vi "listen_can.vi"(10 "reference":refnum<vi>, 11 "队列输入":refnum<queue>) -> ()   [LabVIEW 2018]
uses:
  controls/UI.lvlib
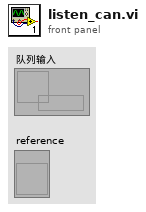
[diagram p1: front panel]
types:
  T1 = typedef "控件 6.ctl" = cluster{"DevType":T2, "Channel":T3, "AccCode":u32, "AccMask":u32, "InitFlag":T4, "Mode":T5, "kBaudRate":u8, "Fliter":T6, "Open":bool, "Close":bool, "连接状态":bool, "SendCnt":u32, "RecvCnt":u32, "Send":bool, "ID":u32, "Data":string, "Type":u8, "Format":u8, "Clear":bool, "list":i32, "路径":path, "RcvEnable":bool}
  T2 = typedef "can库.lvlib/ControlCAN.lvlib/DevType.ctl" = u32
  T3 = typedef "can库.lvlib/ControlCAN.lvlib/CAN Channel.ctl" = u32
  T4 = typedef "can库.lvlib/ControlCAN.lvlib/InitFlag.ctl" = u32
  T5 = typedef "can库.lvlib/ControlCAN.lvlib/Mode.ctl" = u8
  T6 = typedef "can库.lvlib/ControlCAN.lvlib/Fliter.ctl" = u8
  T7 = typedef "Settings.lvlib/Settings.ctl" = cluster{"当前项目UI":T8, "EHA模拟UI":T9, "模拟负载UI":T10, "模拟控制UI":T11, "串口通信UI":T1, "数据记录UI":T12, "控制参数UI":T13, "安全报警UI":T14, "数据显示UI":T15, "硬件配置":T16, "数据显示配置":T18, "串口通信配置":T22, "CAN Status":T24}
  T8 = typedef "控件 5.ctl" = cluster{"控制参数配置":string, "模拟响应配置":string, "串口通信配置":string, "数据显示配置":string, "数据记录配置":string, "安全/报警配置":string, "模拟负载数据":string, "模拟加载数据":string, "总电源":bool, "电机1上电":bool, "电机2上电":bool, "串口连接":bool, "电机1\n相电流报警":bool, "电机2\n相电流报警":bool, "电机1\n母线电压报警":bool, "电机2\n母线电压报警":bool, "保存设置":bool, "从文件加载":bool, "恢复默认设置":bool, "路径":path, "项目路径":path, "项目名":string, "创建时间":string, "上次使用时间":string}
  T9 = typedef "EHA模拟UI.ctl" = cluster{"液压缸有效面积":dbl, "活塞初始位置":dbl, "气体多变系数k":dbl, "柱塞泵口2泄露系数":dbl, "柱塞泵粘性摩擦系数":dbl, "液压缸粘性摩擦系数":dbl, "液压缸有效长度":dbl, "油箱初始压力":dbl, "单向阀通流系数":dbl, "泵口1到口2泄露系数":dbl, "柱塞泵静摩擦力矩":dbl, "液压油体积模量":dbl, "保存设置":bool, "从文件加载":bool, "恢复默认设置":bool, "路径":path, "液压缸内泄露系数":dbl, "油箱气囊初始体积":dbl, "柱塞泵口1泄露系数":dbl, "柱塞泵排量":dbl, "液压缸静摩擦力":dbl, "液压杆到\n液压缸的总质量":dbl}
  T10 = typedef "控件 9.ctl" = cluster{"负载数据":string, "负载数据 2":waveform(dbl)[], "保存设置":bool, "恢复默认设置":bool}
  T11 = typedef "控件 7.ctl" = cluster{"控制数据":string, "负载数据 2":waveform(dbl)[], "保存设置":bool, "恢复默认设置":bool}
  T12 = typedef "控件 3.ctl" = cluster{"保存路径":path, "文件名":string, "后缀":string, "保存格式":string, "复选框":bool, "保存设置":bool, "从文件加载":bool, "恢复默认设置":bool, "路径":path, "TDMS文件引用":refnum<k34>}
  T13 = typedef "控件 1.ctl" = cluster{"d轴电流环P_M":dbl, "转速环P":dbl, "q轴电流环P":dbl, "d轴电流环P":dbl, "转矩环P_M":dbl, "去轴电流环P_M":dbl, "转速环I":dbl, "q轴电流环I":dbl, "d轴电流环I":dbl, "转矩环I_M":dbl, "q轴电流环I_M":dbl, "d轴电流环I_M":dbl, "保存设置":bool, "从文件加载":bool, "恢复默认设置":bool, "路径":path, "位置环P":dbl, "位置环I":dbl, "转速环限幅":dbl, "q轴电流环限幅":dbl, "d轴电流环限幅":dbl, "位置环限幅":dbl, "转矩环限幅_M":dbl, "q轴电流环限幅_M":dbl, "d轴电流环限幅_M":dbl}
  T14 = typedef "控件 4.ctl" = cluster{"报警扭矩":dbl, "过低母线电压":dbl, "过高母线电压":dbl, "母线电流限制":dbl, "相电流报警":dbl, "串口超时报警":dbl, "转速报警":dbl, "过热报警":dbl, "操作":u16, "操作 2":u16, "操作 3":u16, "操作 4":u16, "操作 5":u16, "操作 6":u16, "操作 7":u16, "操作 8":u16, "保存设置":bool, "从文件加载":bool, "恢复默认设置":bool, "路径":path}
  T15 = typedef "控件 2.ctl" = cluster{"保存设置":bool, "从文件加载":bool, "恢复默认设置":bool, "实验":i32, "波形输出":i32, "组件":i32, "曲线":i32, "滤波器":i32, "删除曲线":bool, "清理图像":bool, "添加曲线":bool, "数据选点":bool, "确定按钮":bool, "实时显示":bool, "子图":i32, "显示模式":u16, "路径":path, "删除图像":bool, "创建新图":bool}
  T16 = typedef "Acquisition.lvlib/Hardware Configuration.ctl" = cluster{"硬件引用句柄<替换此项>":string, "信号类型<替换该项>":T17}
  T17 = typedef "Acquisition.lvlib/Signal Type.ctl" = enum16{"Sine Wave", "Square with Noise"}
  T18 = typedef "波形图簇.ctl" = cluster{"波形图数":u32, "波形图数组":T19[], "路径":path}
  T19 = typedef "波形图.ctl" = cluster{"显示模式":u16, "子图数":u32, "子图数组":T20[]}
  T20 = typedef "子图.ctl" = cluster{"子图所有曲线":T21[], "曲线数":u32}
  T21 = typedef "曲线簇.ctl" = cluster{"源":string, "组件":u32, "滤波器":u32}
  T22 = typedef "UI.lvlib/串口通信配置.ctl" = cluster{"DevType":T2, "DevIndex":u32, "CanIndex":T3, "VCI_INIT_CONFIG":T23}
  T23 = typedef "can库.lvlib/ControlCAN.lvlib/VCI_INIT_CONFIG.ctl" = cluster{"AccCode":u32, "AccMask":u32, "InitFlag":T4, "Fliter":T6, "Timing0":u8, "Timing1":u8, "Mode":T5}
  T24 = typedef "UI.lvlib/canstatus.ctl" = cluster{"Open":bool, "SendCnt":u32}
  T25 = typedef "can库.lvlib/ControlCAN.lvlib/VCI_CAN_OBJ.ctl" = cluster{"ID":u32, "TimeStamp":u32, "TimeFlag":u8, "SendType":u8, "RemoteFlag":u8, "ExternFlag":u8, "DataLen":u8, "Data":u8[], "Reserved":u8[]}
  T26 = cluster{"Type":enum16{"接收", "发送"}, "Channel":T3, "Time":timestamp, "VCI_CAN_OBJ":T25}[]
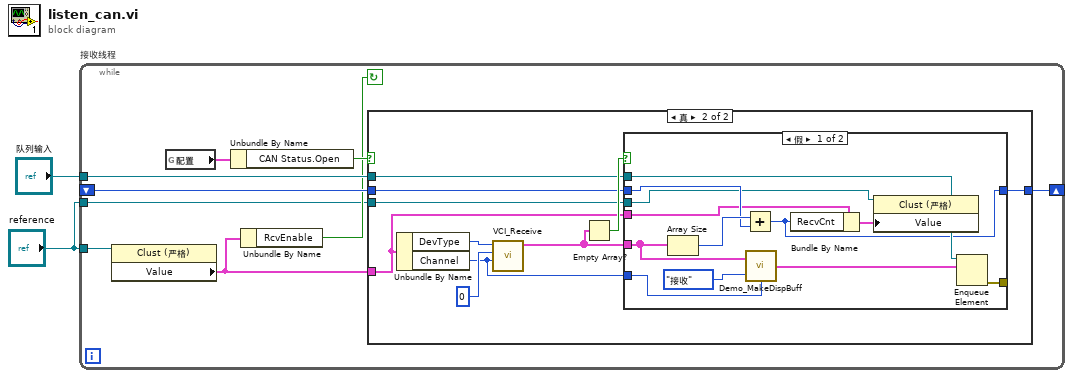
[diagram p0: block diagram]
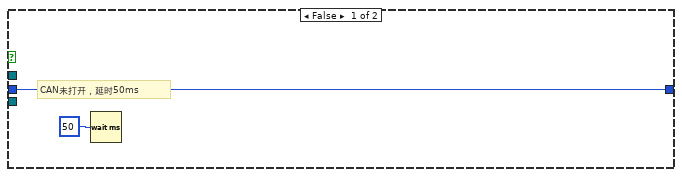
[diagram p2: hidden frame]
diagram:
  n1 = while "接收线程" {
    tunnel: "队列输入" -> [w11]
    shift-right: [w9] -> _
    shift-left: _ -> [w10]
    tunnel: "reference" -> [w4]
    tunnel: "reference" -> [w3]
    stop <- w7 continue-if-true
    n2 = property class="Clust (严格)"(reference=w3) -> ("Value"=w6:T1)  [unwired: 1 in, 2 out]
    n3 = global read "全局配置.vi" "配置"() -> (w5:T7)
    n4 = Unbundle By Name(w5) -> ("CAN Status.Open"=w8:bool)
    n5 = Unbundle By Name(w6) -> ("RcvEnable"=w7:bool)
    n6 = case shown="真" w8 {
      tunnel: w11 -> [_ w20]
      tunnel: w10 -> [w12 w19]
      tunnel: [w12 w18] -> w9
      tunnel: w6 -> [_ w15]
      tunnel: w4 -> [_ w14]
      frame False {
        # "CAN未打开，延时50ms"
        n7 = Wait (ms)(milliseconds to wait=u32 50 ("等待时间（毫秒）")) -> ()  [unwired: 1 out]
      }
      frame True {
        n8 = Unbundle By Name(w15) -> ("DevType"=w17:T2, "Channel"=w16:T3)
        n9 = call "VCI_Receive.vi"("CANIndex"=w16, "DevIndex"=u32 0, "DevType"=w17) -> ("Recieve"=w21:T25[])  [unwired: 3 in, 5 out]
        n10 = Empty Array?(array=w21) -> (empty?=w22:bool)
        n11 = case shown="假" w22 {
          tunnel: w20 -> [w35 _]
          tunnel: w21 -> [w31 _]
          tunnel: [w32 _] -> _
          tunnel: w19 -> [w29 w36]
          tunnel: [w26 w36] -> w18
          tunnel: w16 -> [w28 _]
          tunnel: w15 -> [w25 _]
          tunnel: w14 -> [w24 _]
          frame False {
            n12 = Array Size(array=w31) -> (size(s)=w30:i32)
            n13 = Add(x=w30, y=w29) -> (x+y=w26:i32)
            n14 = call "Demo_MakeDispBuff.vi"("Channel"=w28, "Type"=enum16{"接收", "发送"}."接收", "OBJs"=w31) -> ("Buffer"=w33:T26)
            n15 = Bundle By Name(cluster=w25, "RecvCnt"=w26) -> (w27:T1)
            n16 = property class="Clust (严格)"(reference=w24, "Value"=w27) -> ()  [unwired: 1 in, 2 out]
            n17 = Enqueue Element(queue=w35, element=w33) -> (error out=w32:errorcluster)  [unwired: 1 in, 3 out]
          }
          frame True {
          }
        }
      }
    }
  }
